vi "Process.vi"(8 "error in":errorcluster, 11 "Instrument.Framework-Template in":refnum<class "Instrument.Framework-Template.lvclass">) -> (0 "error out":errorcluster, 3 "Instrument.Framework-Template out":refnum<class "Instrument.Framework-Template.lvclass">)   [LabVIEW 2019, in "Instrument.Framework-Template.lvclass"]
doc: "---------------------------------------------------------------\nJKI State Machine Objects™\nhttp://jki.net/state-machine-objects/\nCopyright (C) 2005-2015, JKI <info@jki.net>\nALL RIGHTS RESERVED"
uses:
  Instrument.Framework-Template.lvclass
  C:/Program Files (x86)/National Instruments/LabVIEW 2019/vi.lib/JKI/JKI SMO/SMO/SMO.lvclass
  C:/Program Files (x86)/National Instruments/LabVIEW 2019/user.lib/LevyLab/Instrument Framework/Instrument/Instrument.lvclass
  Typedefs/PrivateEvents--Framework-Template.MessageToProcess.ctl
  <userlib>/LevyLab/RemoteControl/Typedefs/Message--Cluster.ctl
  Instrument.Framework-Template.lvclass/Instrument.Framework-Template.ctl
  <vilib>/JKI/JKI SMO/SMO/SMO.lvclass/SMO.ctl
  <userlib>/LevyLab/Instrument Framework/Instrument/Typedefs/Instrument.ProtectedCommands--Enum.ctl
  41410b5e-0a7b-4214-bdb2-0ee7b89dae23.vi
  <vilib>/JKI/JKI SMO/SMO/Private/ReftoDVR--SMO.vi
  <vilib>/Utility/Data Type/Get Numeric Information.vi
  <userlib>/LevyLab/Instrument Framework/Instrument/API/Instrument.sendMessageToProcess (string).vi
  <userlib>/LevyLab/Instrument Framework/Instrument Types/SCPI/Instrument.SCPI.lvclass
  <vilib>/JKI/JKI SMO/SMO/SMO.lvclass
  <userlib>/LevyLab/Instrument Framework/Instrument/Instrument.lvclass
  <userlib>/LevyLab/RemoteControl/RemoteControl.lvclass
  C:/Program Files (x86)/National Instruments/LabVIEW 2019/user.lib/LevyLab/Instrument Framework/Instrument Types/SCPI/Instrument.SCPI.lvclass
  <userlib>/LevyLab/Configuration/Debug.lvlib
panel:
  out "Status":string
  out "State History":string
  # "Instrument.Framework-Template"
  # "Framework-Template"
  # "For instructions on how to use the JKI State Machine Objects, examples and video tutorials, visit:\nhttp://jki.net/state-machine-objects/\n\nJKI State Machine Objects™\nhttp://jki.net/state-machine-objects/\nCopyright (C) 2005-2015, JKI <info@jki.net>\nALL RIGHTS RESERVED"
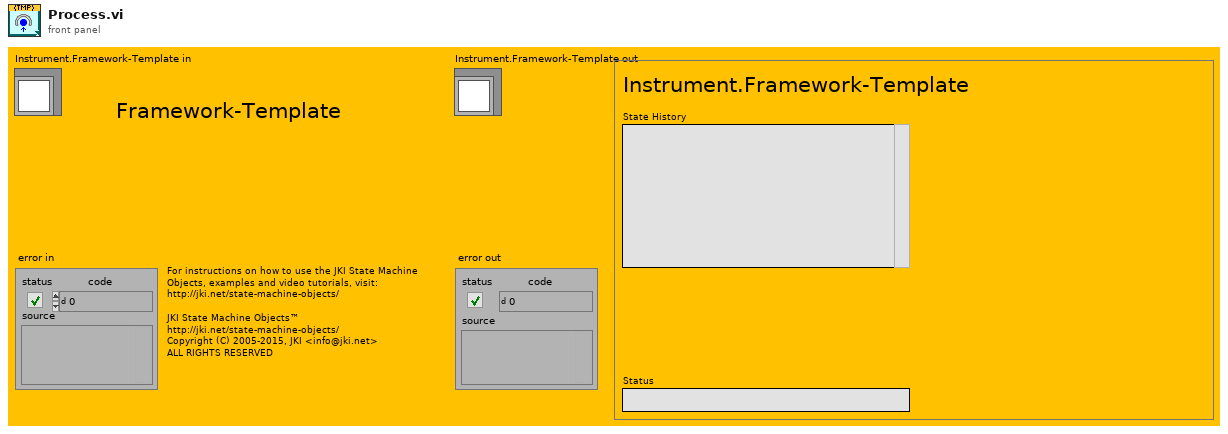
[diagram p1: front panel]
types:
  T1 = enum32{"invalid app kind", "Development System", "Run Time System", "Student Edition", "Embedded LabVIEW", "Evaluation", "Custom"}
  T2 = enum32{"Invalid", "Standard", "Closed", "Hidden", "Minimized", "Maximized"}
  T3 = typedef "Instrument.lvclass/Instrument.ProtectedCommands--Enum.ctl" = enum16{"setConfiguration", "setLogData", "setIDN", "setAll", "setAllData"}
  T4 = typedef "RemoteControl.lvclass/Message--Cluster.ctl" = cluster{"Command":string, "Data":variant, "ID":string}
  T5 = typedef "Instrument.Framework-Template.lvclass/PrivateEvents--Framework-Template.MessageToProcess.ctl" = cluster{"Message":T4}
  T6 = cluster{"Core":cluster{"Current VI Reference":refnum<vi>, "Close Panel on Exit?":bool, "Last Error":cluster{"error":errorcluster, "previous state":string, "remaining states":string}, "Shutdown?":bool}, "SelfRef":refnum<class "Instrument.Framework-Template.lvclass">, "HAL":refnum<class "HAL.lvclass">, "Running Step":i32, "sequence":string[], "MessageToProcess":T5, "UI Behavior":string, "wait":u32}
  T7 = cluster{"Current VI Reference":refnum<vi>, "Close Panel on Exit?":bool, "Last Error":cluster{"error":errorcluster, "previous state":string, "remaining states":string}, "Shutdown?":bool}
  T8 = typedef "Debug.lvlib/Attribute.Debug.lvclass/DebugBehavior.ctl" = enum16{"Normal", "Debug"}
  T9 = typedef "SMO.lvclass/Protected Events.ctl" = cluster{"StopProcesses":refnum<user-event>, "AbortProcesses":refnum<user-event>, "Config Changed":refnum<user-event>, "Dependency":refnum<user-event>}
  T10 = typedef "Instrument.Framework-Template.lvclass/Instrument.Framework-Template.getAll--Cluster.ctl" = cluster{"Levy 1":dbl, "Logger SMO":dbl, "SMO Boolean":bool, "SMO String":string}
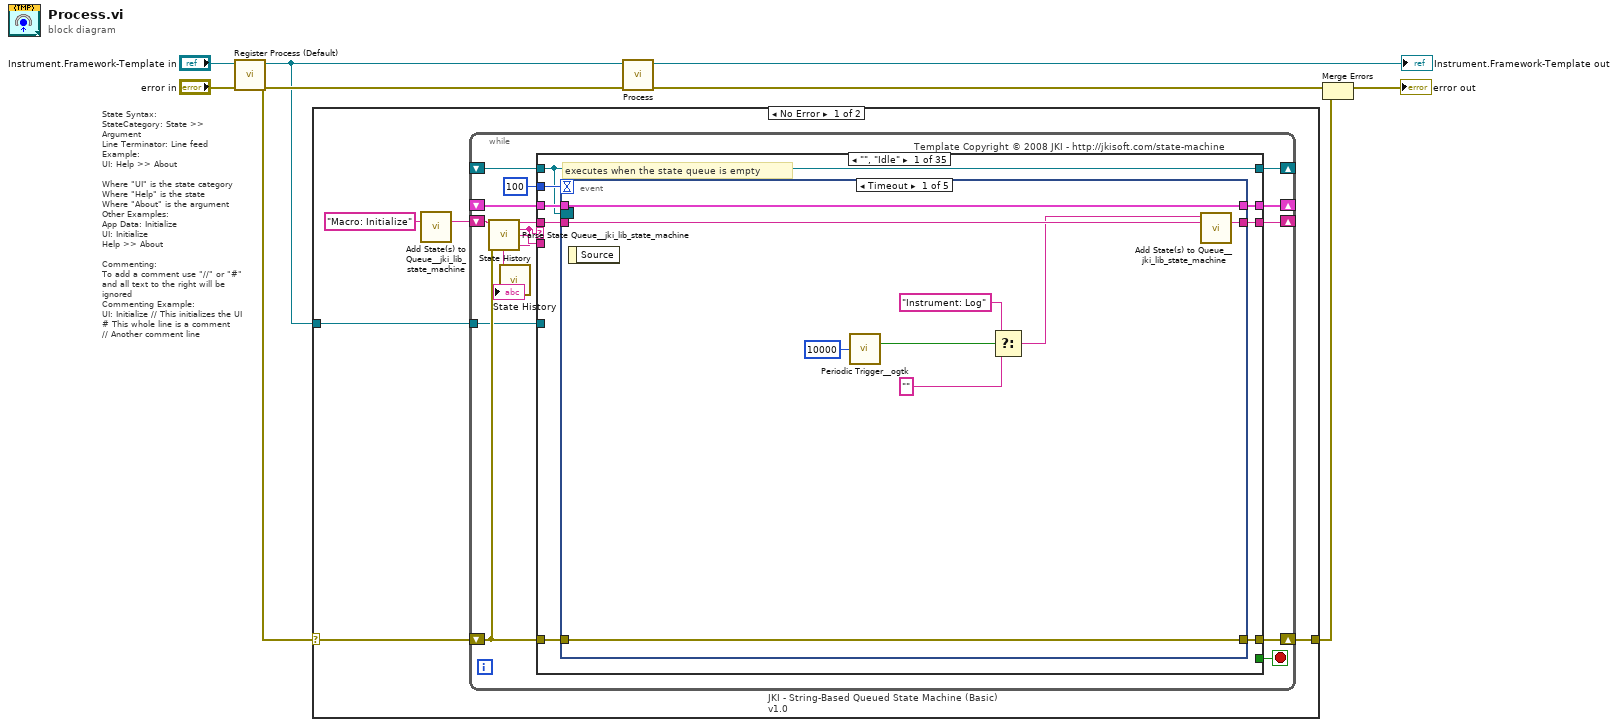
[diagram p0: block diagram]
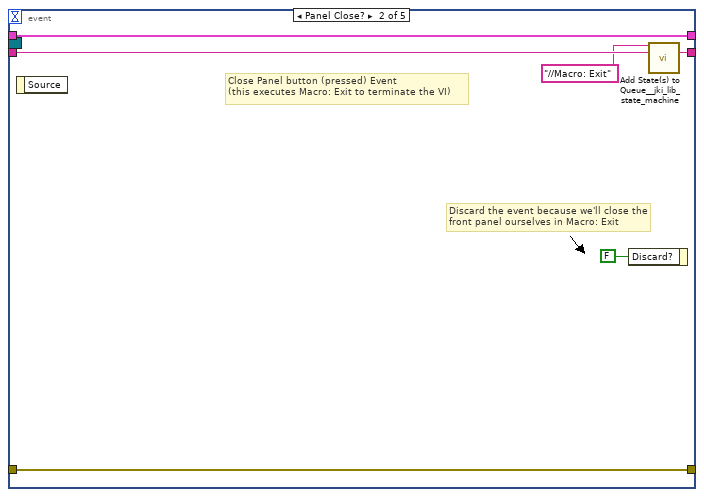
[diagram p2: hidden frame]
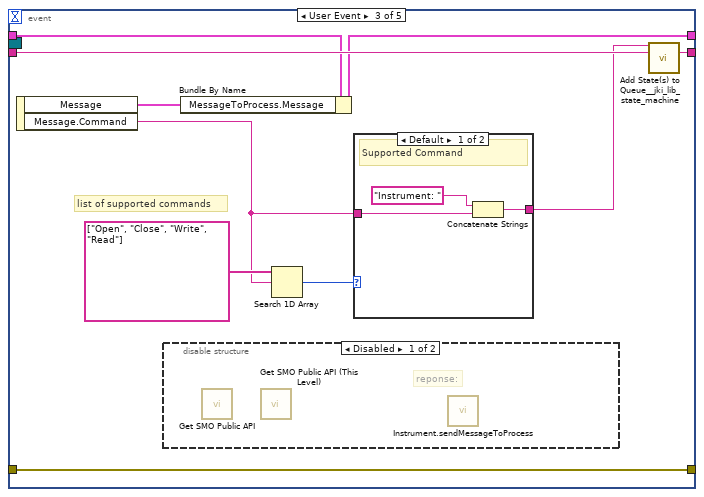
[diagram p3: hidden frame]
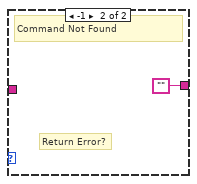
[diagram p5: hidden frame]
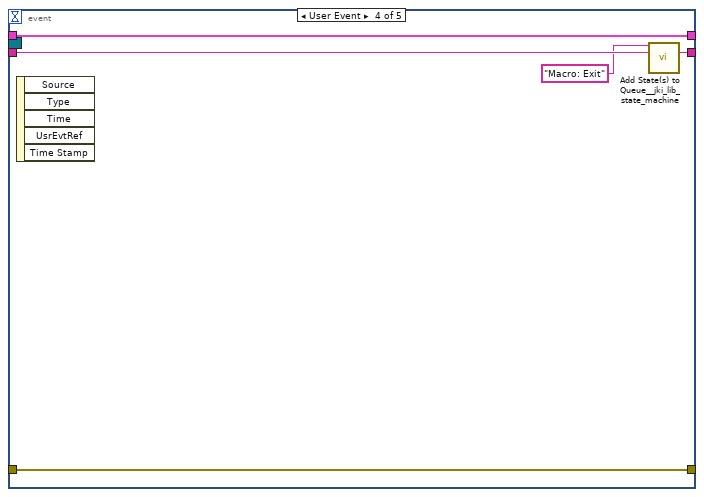
[diagram p6: hidden frame]
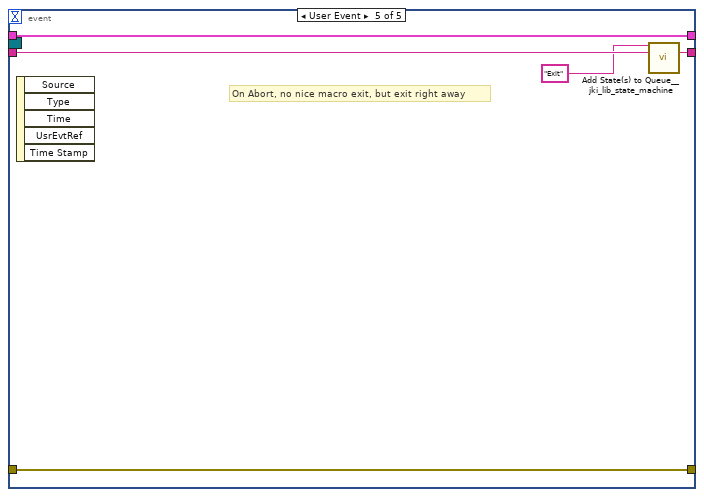
[diagram p7: hidden frame]
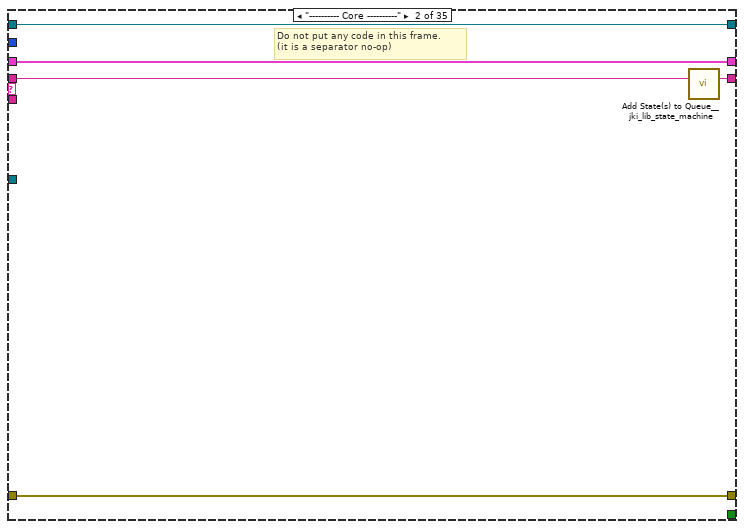
[diagram p8: hidden frame]
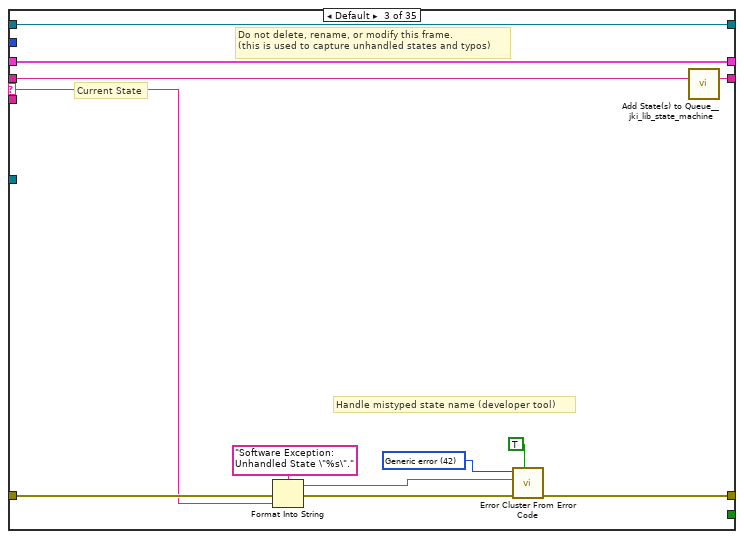
[diagram p9: hidden frame]
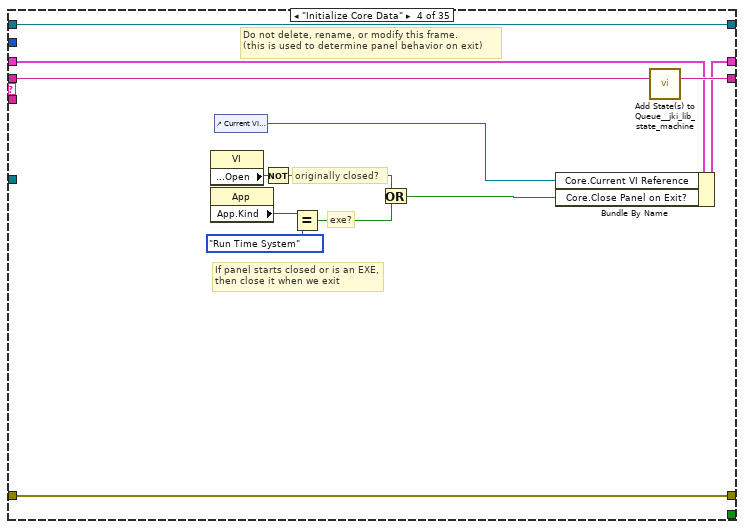
[diagram p10: hidden frame]
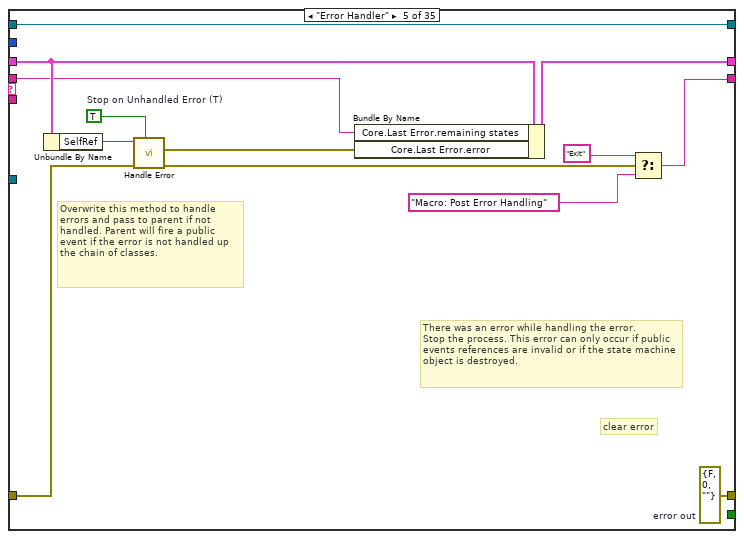
[diagram p11: hidden frame]
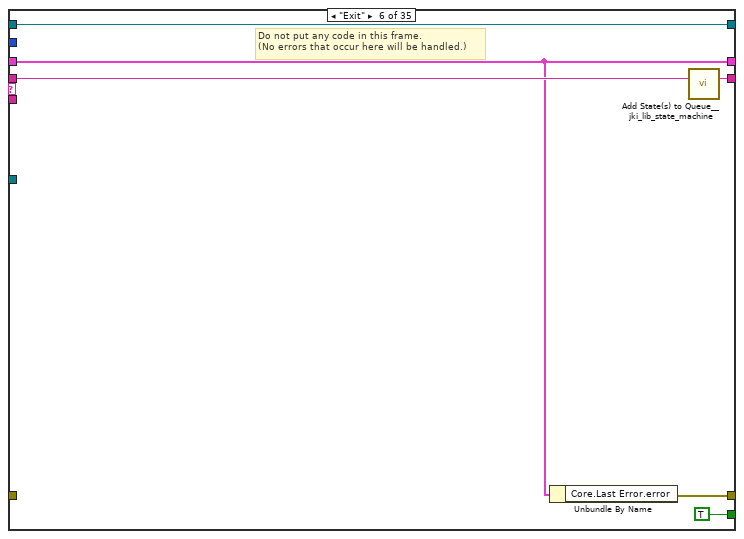
[diagram p12: hidden frame]
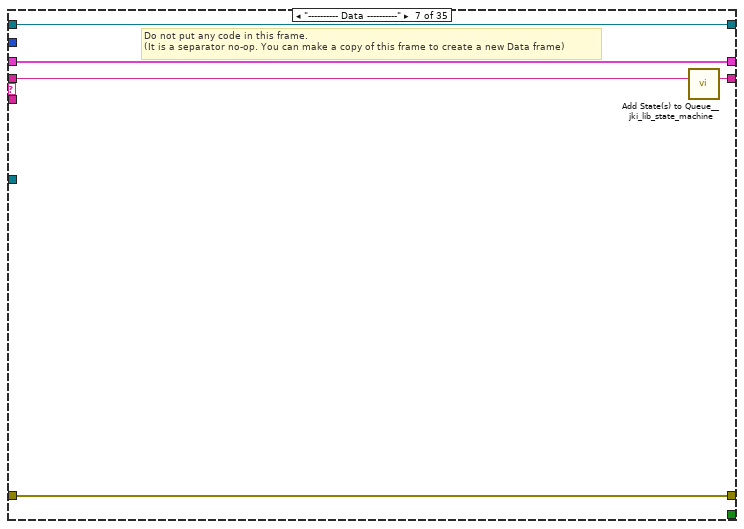
[diagram p13: hidden frame]
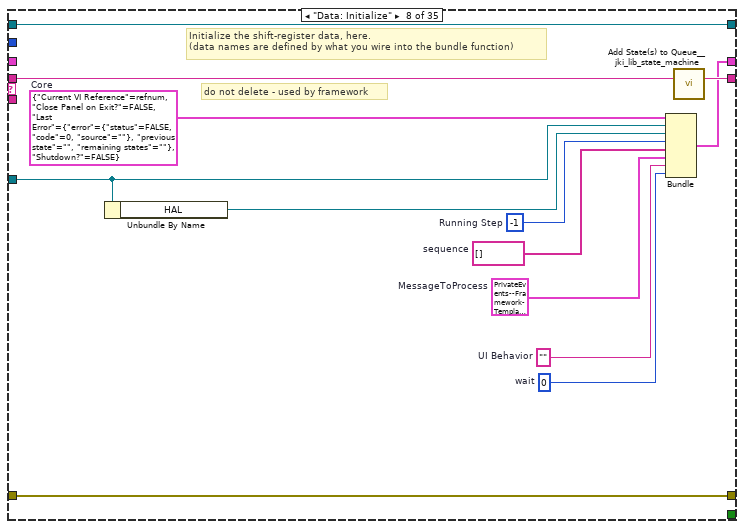
[diagram p14: hidden frame]
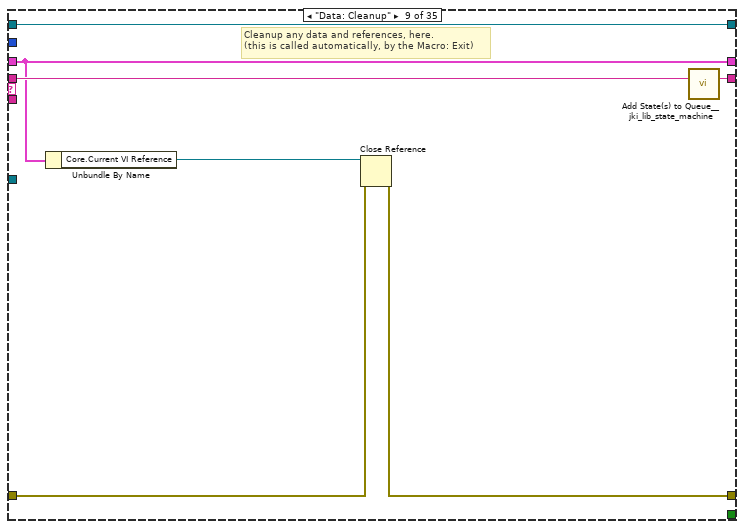
[diagram p15: hidden frame]
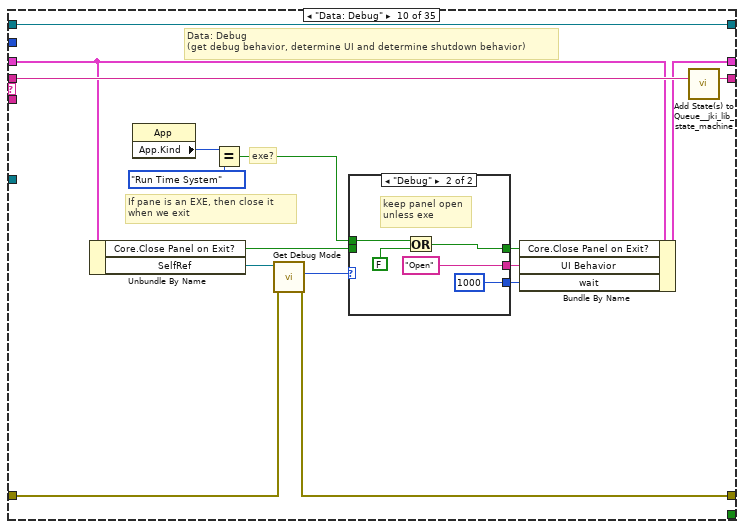
[diagram p16: hidden frame]
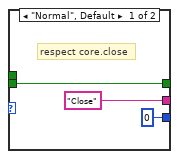
[diagram p17: hidden frame]
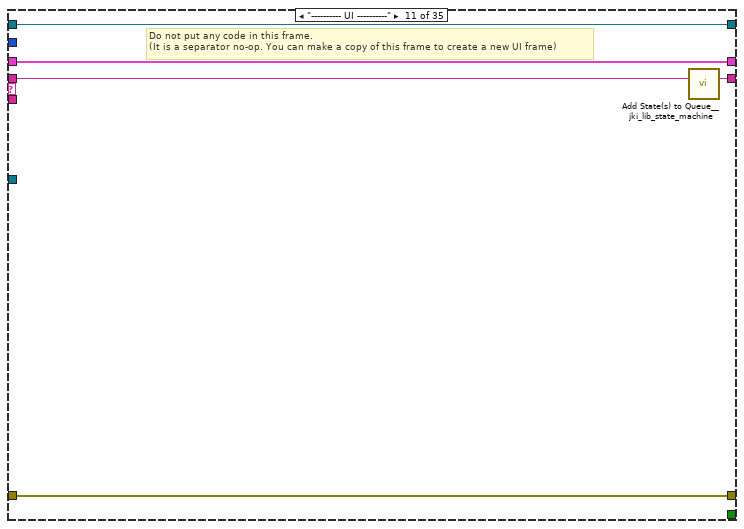
[diagram p18: hidden frame]
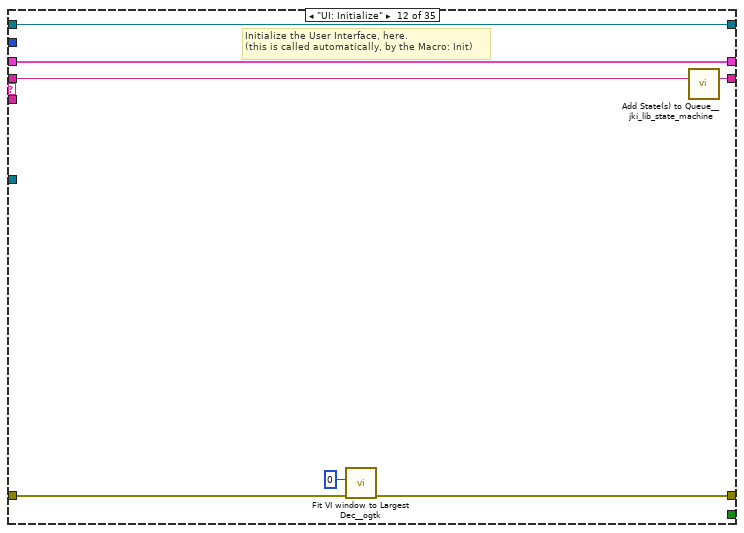
[diagram p19: hidden frame]
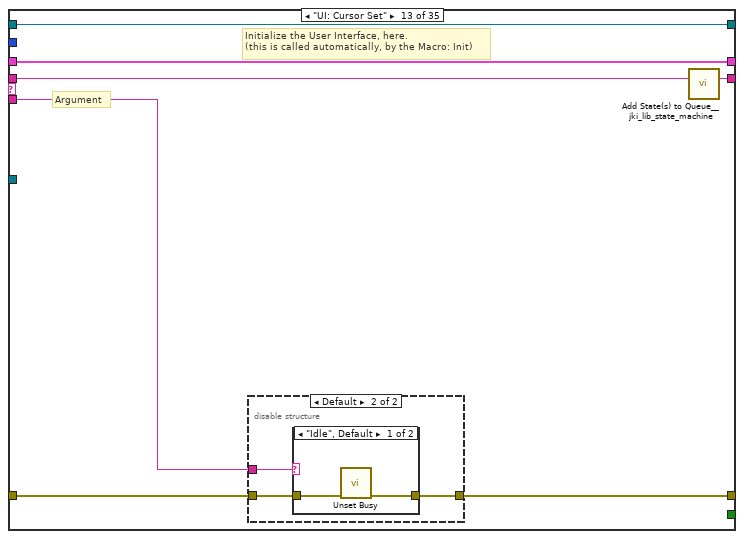
[diagram p20: hidden frame]
diagram:
  # "State Syntax:\nStateCategory: State >> Argument\nLine Terminator: Line feed\nExample:\nUI: Help >> About\n\nWhere \"UI\" is the state category\nWhere \"Help\" is the state\nWhere \"About\" is the argument\nOther Examples:\nApp Data: Initialize\nUI: Initialize\nHelp >> About\n\nCommenting:\nTo add a comment use \"//\" or \"#\" and all text to the right will be ignored\nCommenting Example:\nUI: Initialize // This initializes the UI\n# This whole line is a comment\n// Another comment line"
  n1 = call <vilib>:"Register Process (Default).vi"("error in (no error)"="error in", "SMO"="Instrument.Framework-Template in") -> ("error out"=w5:errorcluster, "SelfRef"=w4:refnum<class "Instrument.Framework-Template.lvclass">)  [unwired: 8 in]
  n2 = case shown="No Error" w5 {
    selector: w5 -> [w10 w459]
    tunnel: w4 -> [w11 _]
    tunnel: [w9 w459] -> w1
    frame No Error {
      n3 = call <vilib>:"Add State(s) to Queue__jki_lib_state_machine.vi"("State(s) in (\"\")"="Macro: Initialize") -> ("States Out"=w13:string)  [unwired: 14 in]
      n4 = while "JKI - String-Based Queued State Machine (Basic) v1.0" {
        shift-right: [w22] -> _
        shift-left: _ -> [w21]
        shift-right: [w25] -> w9
        shift-left: w10 -> [w19]
        shift-right: [w24] -> _
        shift-left: w13 -> [w26]
        tunnel: w11 -> [w18]
        shift-right: [w17] -> _
        shift-left: _ -> [w16]
        stop <- w23 stop-if-true
        # "Template Copyright © 2008 JKI - http://jkisoft.com/state-machine"
        n5 = call <vilib>:"Parse State Queue__jki_lib_state_machine.vi"("State Queue"=w26, "Error In (no error)"=w19) -> ("Remaining States"=w28:string, "Current State"=w15:string, "Arguments"=w27:string)  [unwired: 11 in]
        n6 = call <userlib>:"State History.vi"("Current State"=w15) -> ("History"=→"State History":string)  [unwired: 10 in]
        n7 = case shown="\"\", \"Idle\"" w15 {
          selector: w15 -> [_ _ w82 _ _ _ _ _ _ _ _ _ _ _ _ _ _ _ _ _ _ _ _ _ _ _ _ _ _ _ _ _ _ _ _]
          tunnel: w28 -> [w36 w80 w86 w105 w110 w124 w129 w142 w149 w165 w178 w185 w192 w208 w240 w249 w261 w282 w290 w305 w310 w321 w326 w339 w345 w353 w362 w371 w381 w390 w405 w428 w433 w439 w458]
          tunnel: w27 -> [_ _ _ _ _ _ _ _ _ _ _ _ w186 w202 _ _ _ _ _ _ _ _ _ _ _ _ _ _ _ _ _ _ _ w434 w442]
          tunnel: w21 -> [w34 w77 w84 w96 w114 w120 w126 _ w144 w152 w175 w183 w190 w204 w237 w246 w251 w272 w284 w294 w307 w318 w323 w332 w343 w348 w358 w367 w377 w386 w401 w424 w429 w435 w448]
          tunnel: [w33 w78 w88 w102 w115 w119 w127 w132 w145 w151 w176 w180 w187 w205 w238 w241 w259 w280 w288 w292 w308 w312 w324 w335 w341 w350 w354 w366 w376 w385 w395 w422 w430 w436 w450] -> w25
          tunnel: w19 -> [w32 w78 w87 w102 w116 _ w127 w132 w146 w150 w176 w179 w188 w206 w238 w241 w259 w280 w288 w292 w308 w313 w324 w329 w341 w350 w357 w365 w375 w384 w399 w417 w430 w436 w444]
          tunnel: [w35 w79 w85 w104 w106 w123 w128 w141 w148 w164 w177 w184 w191 w207 w239 w248 w260 w281 w289 w304 w309 w320 w325 w338 w344 w352 w361 w370 w380 w389 w404 w427 w432 w438 w457] -> w24
          tunnel: [_ _ _ _ _ TRUE _ _ _ _ _ _ _ _ _ _ _ _ _ _ _ _ _ _ _ _ _ _ _ _ _ _ _ _ _] -> w23
          tunnel: [w31 w77 w84 w103 w113 w120 w126 w140 w144 w153 w175 w183 w190 w204 w237 w246 w252 w273 w284 w294 w307 w318 w323 w332 w343 w349 w359 w368 w378 w387 w402 w425 w429 w435 w447] -> w22
          tunnel: 100 ("Timeout") -> [w30 _ _ _ _ _ _ _ _ _ _ _ _ _ _ _ _ _ _ _ _ _ _ _ _ _ _ _ _ _ _ _ _ _ _]
          tunnel: w18 -> [_ _ _ _ _ _ _ w133 _ _ _ _ _ _ _ _ _ _ _ _ _ _ _ _ _ _ _ _ _ _ _ _ _ _ _]
          tunnel: [w29 w76 w81 w93 w118 w121 w125 w139 w143 w163 w174 w182 w189 w201 w236 w247 w258 w279 w287 w299 w306 w319 w322 w337 w342 w351 w360 w369 w379 w388 w403 w426 w431 w437 w456] -> w17
          tunnel: w16 -> [w29 w76 w81 w93 w118 w121 w125 w139 w143 w163 w174 w182 w189 w201 w236 w247 w258 w279 w287 w299 w306 w319 w322 _ w342 w351 w360 w369 w379 w388 w403 w426 w431 w437 w456]
          frame "", "Idle" {
            # "executes when the state queue is empty"
            n8 = event shown="[0] Timeout" {
              selector: w29 -> [_ _ _ _ _]
              dyn-events: _ -> [_ _ _ _ _]
              timeout: w30 -> [_ _ _ _ _]
              tunnel: w36 -> [w45 w51 w61 w70 w75]
              tunnel: [w44 w50 w60 w69 w74] -> w35
              tunnel: w34 -> [w42 w48 w53 w67 w72]
              tunnel: [w43 w49 w59 w68 w73] -> w33
              tunnel: w32 -> [w43 w49 w59 w68 w73]
              tunnel: [w42 w48 w54 w67 w72] -> w31
              event Timeout {
                n9 = event-data() -> ()  [unwired: 1 in, 1 out]
                n10 = call <userlib>:"Periodic Trigger__ogtk.vi"("time (ms)"=u32 10000) -> ("Triggered"=w39:bool)  [unwired: 12 in, 2 out]
                n11 = Select(t="Instrument: Log", s=w39, f="") -> (s? t:f=w40:string)
                n12 = call <vilib>:"Add State(s) to Queue__jki_lib_state_machine.vi"("State(s) in Front (\"\")"=w40, "State(s) in (\"\")"=w45) -> ("States Out"=w44:string)  [unwired: 13 in]
              }
              event Panel Close? {
                # "Discard the event because we'll close the front panel ourselves in Macro: Exit"
                # "Close Panel button (pressed) Event\n(this executes Macro: Exit to terminate the VI)"
                n13 = event-data() -> ()  [unwired: 1 in, 1 out]
                n14 = event-data("Discard?"=FALSE) -> ()  [unwired: 1 in, 1 out]
                n15 = call <vilib>:"Add State(s) to Queue__jki_lib_state_machine.vi"("State(s) in Front (\"\")"="//Macro: Exit", "State(s) in (\"\")"=w51) -> ("States Out"=w50:string)  [unwired: 13 in]
              }
              event User Event {
                # "list of supported commands"
                n16 = event-data() -> ("Message"=w52:T4, "Message.Command"=w55:string)  [unwired: 1 in]
                n17 = disable-structure shown="Disabled" {
                  frame Disabled {
                    # "reponse:"
                    n18 = call-dynamic "Get SMO Public API.vi"() -> ()  [unwired: 9 in, 3 out]
                    n19 = call-dynamic "Get SMO Public API (This Level).vi"() -> ()  [unwired: 9 in, 3 out]
                    n20 = call-poly <userlib>:"Instrument.sendMessageToProcess.vi"() -> ()  [unwired: 10 in, 2 out]
                  }
                  frame Enabled {
                  }
                }
                n21 = Bundle By Name(cluster=w53, "MessageToProcess.Message"=w52) -> (w54:T6)
                n22 = Search 1D Array(1D array=string[] ["Open", "Close", "Write", "Read"], element=w55) -> (index of element=w58:i32)  [unwired: 1 in]
                n23 = case shown="Default" w58 {
                  tunnel: [w64 ""] -> w56
                  tunnel: w55 -> [w63 _]
                  frame Default {
                    # "Supported Command"
                    n24 = Concatenate Strings("Instrument: ", w63) -> (w64:string)
                  }
                  frame -1 {
                    # "Return Error?"
                    # "Command Not Found"
                  }
                }
                n25 = call <vilib>:"Add State(s) to Queue__jki_lib_state_machine.vi"("State(s) in Front (\"\")"=w56, "State(s) in (\"\")"=w61) -> ("States Out"=w60:string)  [unwired: 13 in]
              }
              event User Event {
                n26 = event-data() -> ()  [unwired: 1 in, 5 out]
                n27 = call <vilib>:"Add State(s) to Queue__jki_lib_state_machine.vi"("State(s) in Front (\"\")"="Macro: Exit", "State(s) in (\"\")"=w70) -> ("States Out"=w69:string)  [unwired: 13 in]
              }
              event User Event {
                # "On Abort, no nice macro exit, but exit right away"
                n28 = event-data() -> ()  [unwired: 1 in, 5 out]
                n29 = call <vilib>:"Add State(s) to Queue__jki_lib_state_machine.vi"("State(s) in Front (\"\")"="Exit", "State(s) in (\"\")"=w75) -> ("States Out"=w74:string)  [unwired: 13 in]
              }
            }
          }
          frame "---------- Core ----------" {
            # "Do not put any code in this frame.\n(it is a separator no-op)"
            n30 = call <vilib>:"Add State(s) to Queue__jki_lib_state_machine.vi"("State(s) in (\"\")"=w80) -> ("States Out"=w79:string)  [unwired: 14 in]
          }
          frame Default {
            w91 = 42 items=["No error", "Argument error", "Memory is full", "Out of zone", "End of file", "File already open", "Generic file I/O error", "File not found", "File permission error", "Disk is full", "Duplicate path", "Too many files open", "System feature not enabled", "Resource file not found", "Cannot add resource", "Resource not found", "Image not found", "Image memory error", "Pen does not exist", "Config type invalid", "Config token not found", "Config parse error", "Config memory error", "Bad external code format", "Bad external code offset", "External code not present", "Null window", "Destroy window error", "Null menu", "Print aborted", "Bad print record", "Print driver error", "Windows error during printing", "Memory error during printing", "Print dialog error", "Generic print error", "Invalid device refnum", "Device not found", "Device parameter error", "Device unit error", "Cannot open device", "Device call aborted", "Generic error", "Cancelled by user", "Object ID too low", "Object ID too high", "Object not in heap", "Unknown heap", "Unknown object (invalid DefProc)", "Unknown object (DefProc not in table)", "Message out of range", "Invalid (null) method", "Unknown message", "Manager call not supported", "Bad address", "Network operation in progress", "Network operation timed out", "Connection is busy", "Network attribute not supported", "Network error", "Address in use", "System out of memory", "Connection aborted", "Connection refused", "Not connected", "Already connected", "Connection closed", "Initialization error (interapplication manager)", "Bad occurrence", "Wait on unbound occurrence handler", "Occurrence queue overflow", "Datalog type conflict", "Unused", "Unrecognized type (interapplication manager)", "Memory corrupt", "Failed to make temporary DLL", "Old CIN version", "Drag socket not found", "Failed to load drop-object", "Failed to register OLE object", "Failed to release OLE object", "Format specifier type mismatch", "Unknown format specifier", "Too few format specifiers", "Too many format specifiers", "Scan failed", "Newer CIN version", "Error converting to variant", "Runtime menu error", "Password tampered", "Variant attribute not found", "Incompatible variant data type", "Event data is not available", "Event Store is not present", "Occurrence is not found", "Event Queue is not created", "Event info is not available", "Refnum passed is NULL", "Error retrieving Class GUID", "Error retrieving CoClass GUID", "Error retrieving TypeLib GUID.", "Bad built application magic bytes.", "Specific driver is different from the specific driver associated with the Logical Name.", "There is no session opened to the class driver.", "Max Error", "MAX - Error with config objects", "MAX - Error loading configuration", "MAX - Group not supported"]
            # "Current State"
            # "Do not delete, rename, or modify this frame.\n(this is used to capture unhandled states and typos)"
            # "Handle mistyped state name (developer tool)"
            n31 = Format Into String(format string="Software Exception: Unhandled State \"%s\"." ("message"), error in=w87, w82) -> (resulting string=w90:string, error out=w89:errorcluster)  [unwired: 1 in]
            n32 = call <vilib>:"Error Cluster From Error Code.vi"("show call chain? (False)"=TRUE, "error in (no error)"=w89, "error message (\"\")"=w90, "error code (0)"=w91) -> ("error out"=w88:errorcluster)  [unwired: 5 in]
            n33 = call <vilib>:"Add State(s) to Queue__jki_lib_state_machine.vi"("State(s) in (\"\")"=w86) -> ("States Out"=w85:string)  [unwired: 14 in]
          }
          frame "Initialize Core Data" {
            # "Do not delete, rename, or modify this frame.\n(this is used to determine panel behavior on exit)"
            # "originally closed?"
            # "exe?"
            # "If panel starts closed or is an EXE, then close it when we exit"
            n34 = property class="VI"() -> ("Front Panel.Open"=w101:bool)  [unwired: 2 in, 2 out]
            n35 = property class="App"() -> ("App.Kind"=w100:T1)  [unwired: 2 in, 2 out]
            n36 = control-ref of="Current VI Reference"() -> (w94:refnum<vi>)
            n37 = Not(x=w101) -> (.not. x?=w98:bool)
            n38 = Equal?(x=w100, y=T1."Run Time System" ("Application:Kind")) -> (x = y?=w97:bool)
            n39 = Or(x=w98, y=w97) -> (x .or. y?=w95:bool)
            n40 = Bundle By Name(cluster=w96, "Core.Current VI Reference"=w94, "Core.Close Panel on Exit?"=w95) -> (w103:T6)
            n41 = call <vilib>:"Add State(s) to Queue__jki_lib_state_machine.vi"("State(s) in (\"\")"=w105) -> ("States Out"=w104:string)  [unwired: 14 in]
          }
          frame "Error Handler" {
            w111 = TRUE  # Stop on Unhandled Error (T)
            w115 = errorcluster {"status"=FALSE, "code"=0, "source"=""}  # error out
            # "clear error"
            # "There was an error while handling the error.\nStop the process. This error can only occur if public events references are invalid or if the state machine object is destroyed."
            # "Overwrite this method to handle errors and pass to parent if not handled. Parent will fire a public event if the error is not handled up the chain of classes."
            n42 = Unbundle By Name(w114) -> ("SelfRef"=w117:refnum<class "Instrument.Framework-Template.lvclass">)
            n43 = call-dynamic "Handle Error.vi"("Stop on Unhandled Error (T)"=w111, "error in"=w116, "SMO"=w117) -> ("handling error"=w107:errorcluster, "Unhandled error"=w112:errorcluster)  [unwired: 6 in, 1 out]
            n44 = Bundle By Name(cluster=w114, "Core.Last Error.remaining states"=w110, "Core.Last Error.error"=w112) -> (w113:T6)
            n45 = Select(t="Exit", s=w107, f="Macro: Post Error Handling") -> (s? t:f=w106:string)
          }
          frame "Exit" {
            # "Do not put any code in this frame.\n(No errors that occur here will be handled.)"
            n46 = Unbundle By Name(w120) -> ("Core.Last Error.error"=w119:errorcluster)
            n47 = call <vilib>:"Add State(s) to Queue__jki_lib_state_machine.vi"("State(s) in (\"\")"=w124) -> ("States Out"=w123:string)  [unwired: 14 in]
          }
          frame "---------- Data ----------" {
            # "Do not put any code in this frame.\n(It is a separator no-op. You can make a copy of this frame to create a new Data frame)"
            n48 = call <vilib>:"Add State(s) to Queue__jki_lib_state_machine.vi"("State(s) in (\"\")"=w129) -> ("States Out"=w128:string)  [unwired: 14 in]
          }
          frame "Data: Initialize" {
            w130 = u32 0  # wait
            w131 = ""  # UI Behavior
            w135 = T5 {"Message"={"Command"="", "Data"=variant(string ""), "ID"=""}}  # MessageToProcess
            w136 = string[] []  # sequence
            w137 = -1  # Running Step
            w138 = T7 {"Current VI Reference"=refnum, "Close Panel on Exit?"=FALSE, "Last Error"={"error"={"status"=FALSE, "code"=0, "source"=""}, "previous state"="", "remaining states"=""}, "Shutdown?"=FALSE}  # Core
            # "do not delete - used by framework"
            # "Initialize the shift-register data, here.\n(data names are defined by what you wire into the bundle function)"
            n49 = Unbundle By Name(w133) -> ("HAL"=w134:refnum<class "HAL.lvclass">)
            n50 = Bundle("Core"=w138, "SelfRef"=w133, "HAL"=w134, "Running Step"=w137, "sequence"=w136, "MessageToProcess"=w135, "UI Behavior"=w131, "wait"=w130) -> (w140:T6)  [unwired: 1 in]
            n51 = call <vilib>:"Add State(s) to Queue__jki_lib_state_machine.vi"("State(s) in (\"\")"=w142) -> ("States Out"=w141:string)  [unwired: 14 in]
          }
          frame "Data: Cleanup" {
            # "Cleanup any data and references, here.\n(this is called automatically, by the Macro: Exit)"
            n52 = Unbundle By Name(w144) -> ("Core.Current VI Reference"=w147:refnum<vi>)
            n53 = Close Reference(reference=w147, error in (no error)=w146) -> (error out=w145:errorcluster)
            n54 = call <vilib>:"Add State(s) to Queue__jki_lib_state_machine.vi"("State(s) in (\"\")"=w149) -> ("States Out"=w148:string)  [unwired: 14 in]
          }
          frame "Data: Debug" {
            # "exe?"
            # "If pane is an EXE, then close it when we exit"
            # "Data: Debug\n(get debug behavior, determine UI and determine shutdown behavior)"
            n55 = Unbundle By Name(w152) -> ("Core.Close Panel on Exit?"=w155:bool, "SelfRef"=w162:refnum<class "Instrument.Framework-Template.lvclass">)
            n56 = property class="App"() -> ("App.Kind"=w158:T1)  [unwired: 2 in, 2 out]
            n57 = Equal?(x=w158, y=T1."Run Time System" ("Application:Kind")) -> (x = y?=w154:bool)
            n58 = call <userlib>:"Get Debug Mode.vi"("error in (no error)"=w150, "SMO"=w162) -> ("error out"=w151:errorcluster, "Behavior"=w161:T8)  [unwired: 7 in, 1 out]
            n59 = case shown="\"Debug\"" w161 {
              tunnel: ["Close" "Open"] -> w160
              tunnel: [u32 0 ("wait") u32 1000 ("wait")] -> w159
              tunnel: [w166 w169] -> w156
              tunnel: w155 -> [w166 _]
              tunnel: w154 -> [_ w171]
              frame "Normal", Default {
                # "respect core.close"
              }
              frame "Debug" {
                # "keep panel open\nunless exe"
                n60 = Or(x=w171, y=FALSE) -> (x .or. y?=w169:bool)
              }
            }
            n61 = Bundle By Name(cluster=w152, "Core.Close Panel on Exit?"=w156, "UI Behavior"=w160, "wait"=w159) -> (w153:T6)
            n62 = call <vilib>:"Add State(s) to Queue__jki_lib_state_machine.vi"("State(s) in (\"\")"=w165) -> ("States Out"=w164:string)  [unwired: 14 in]
          }
          frame "---------- UI ----------" {
            # "Do not put any code in this frame.\n(It is a separator no-op. You can make a copy of this frame to create a new UI frame)"
            n63 = call <vilib>:"Add State(s) to Queue__jki_lib_state_machine.vi"("State(s) in (\"\")"=w178) -> ("States Out"=w177:string)  [unwired: 14 in]
          }
          frame "UI: Initialize" {
            # "Initialize the User Interface, here.\n(this is called automatically, by the Macro: Init)"
            n64 = call <userlib>:"Fit VI window to Largest Dec__ogtk.vi"("error in (no error)"=w179, "border spacing (2 px)"=0) -> ("error out"=w180:errorcluster)  [unwired: 4 in, 1 out]
            n65 = call <vilib>:"Add State(s) to Queue__jki_lib_state_machine.vi"("State(s) in (\"\")"=w185) -> ("States Out"=w184:string)  [unwired: 14 in]
          }
          frame "UI: Cursor Set" {
            # "Argument"
            # "Initialize the User Interface, here.\n(this is called automatically, by the Macro: Init)"
            n66 = disable-structure shown="Default" {
              disable-tunnel: w188 -> [w193 w196]
              disable-tunnel: [w193 w195] -> w187
              disable-tunnel: w186 -> [_ w194]
              frame condition #0 {
              }
              frame condition #1 (active) {
                n67 = case shown="\"Idle\", Default" w194 {
                  tunnel: w196 -> [w198 w200]
                  tunnel: [w197 w199] -> w195
                  frame "Idle", Default {
                    n68 = call <vilib>:"Unset Busy.vi"("error in (no error)"=w198) -> ("error out"=w197:errorcluster)  [unwired: 10 in]
                  }
                  frame "Busy" {
                    n69 = call <vilib>:"Set Busy.vi"("error in (no error)"=w200) -> ("error out"=w199:errorcluster)  [unwired: 9 in, 1 out]
                  }
                }
              }
            }
            n70 = call <vilib>:"Add State(s) to Queue__jki_lib_state_machine.vi"("State(s) in (\"\")"=w192) -> ("States Out"=w191:string)  [unwired: 14 in]
          }
          frame "UI: Front Panel State" {
            # "Argument"
            # "Set Front Panel Open or Closed\n(Usage: \"UI: Front Panel State >> Open|Close\")"
            n71 = Unbundle By Name(w204) -> ("Core.Current VI Reference"=w203:refnum<vi>)
            n72 = disable-structure shown="TARGET_TYPE==RT" {
              disable-tunnel: w206 -> [w212 w235]
              disable-tunnel: [w211 w235] -> w205
              disable-tunnel: w203 -> [w210 _]
              disable-tunnel: w202 -> [w209 _]
              frame condition #0 (active) {
                n73 = case shown="\"Close\"" w209 {
                  tunnel: w212 -> [w216 w229]
                  tunnel: [w218 w230] -> w211
                  tunnel: w210 -> [w217 w227]
                  frame "Open", Default {
                    n74 = property class="VI"(reference=w217, error in=w216) -> (reference out=w214:refnum<vi>, error out=w215:errorcluster, "FP.State"=w213:T2)
                    n75 = case shown="\"Closed\"" w213 {
                      tunnel: [w221 w224] -> w218
                      tunnel: w215 -> [w220 w224]
                      tunnel: w214 -> [w219 _]
                      frame "Closed" {
                        n76 = invoke class="VI" method="FP.Open"(reference=w219, error in=w220, "Activate"=TRUE, "State"=T2."Standard") -> (error out=w221:errorcluster)  [unwired: 1 in, 4 out]
                      }
                      frame Default {
                      }
                    }
                  }
                  frame "Close" {
                    n77 = property class="VI"(reference=w227, error in=w229) -> (reference out=w226:refnum<vi>, error out=w228:errorcluster, "FP.State"=w225:T2)
                    n78 = case shown="Default" w225 {
                      tunnel: [w231 w234] -> w230
                      tunnel: w228 -> [w231 w233]
                      tunnel: w226 -> [_ w232]
                      frame "Invalid", "Closed" {
                      }
                      frame Default {
                        n79 = invoke class="VI" method="FP.Close"(reference=w232, error in=w233) -> (error out=w234:errorcluster)  [unwired: 1 in, 2 out]
                      }
                    }
                  }
                }
              }
              frame condition #1 {
              }
            }
            n80 = call <vilib>:"Add State(s) to Queue__jki_lib_state_machine.vi"("State(s) in (\"\")"=w208) -> ("States Out"=w207:string)  [unwired: 14 in]
          }
          frame "---------- Macro ----------" {
            # "Do not put any code in this frame.\n(It is a separator no-op. You can make a copy of this frame to create a new Macro frame)"
            n81 = call <vilib>:"Add State(s) to Queue__jki_lib_state_machine.vi"("State(s) in (\"\")"=w240) -> ("States Out"=w239:string)  [unwired: 14 in]
          }
          frame "Macro: Initialize" {
            # "Initialization Macro\n(This is called once, when the VI starts)"
            n82 = call <vilib>:"Add State(s) to Queue__jki_lib_state_machine.vi"("State(s) in Front (\"\")"="Data: Initialize\nInitialize Core Data\nEvents: Register", "State(s) in (\"\")"="Process: Sync", "State(s) at Back (\"\")"="UI: Initialize\nUI: Front Panel State >> Close\nInstrument: Open\nMacro: Debug") -> ("States Out"=w244:string)  [unwired: 12 in]
            n83 = call <vilib>:"Add State(s) to Queue__jki_lib_state_machine.vi"("State(s) in Front (\"\")"=w244, "State(s) in (\"\")"=w249) -> ("States Out"=w248:string)  [unwired: 13 in]
          }
          frame "Macro: Post Error Handling" {
            # "Clear Last Error?"
            n84 = Unbundle By Name(w251) -> ("Core.Last Error.remaining states"=w253:string, "Core.Shutdown?"=w254:bool)
            n85 = Unbundle By Name(w251) -> ("Core.Last Error.error"=w257:errorcluster)
            n86 = case shown="False" FALSE {
              tunnel: w257 -> [w265 _]
              tunnel: [w265 _] -> w256
              frame False {
              }
              frame True {
              }
            }
            n87 = case shown="False" w254 {
              tunnel: w253 -> [w262 w264]
              tunnel: [w262 w263] -> w250
              frame False {
                # "These are the remaining states (at the moment the error occured). States can be altered according to business logic."
                # "NOT SHUTTING DOWN"
              }
              frame True {
                # "Developer can decide to alter the states but should be aware that during the shutdown process, there are certain states that must be run for the SMO to properly shut itself (and this process) down. As such, one can add states to perform additional clean-ups, but should append the remaining state to be executed."
                # "SHUTTING DOWN"
                n88 = call <vilib>:"Add State(s) to Queue__jki_lib_state_machine.vi"("State(s) in (\"\")"=w264) -> ("States Out"=w263:string)  [unwired: 14 in]
              }
            }
            n89 = Bundle By Name(cluster=w251, "Core.Last Error.error"=w256) -> (w252:T6)
            n90 = call <vilib>:"Add State(s) to Queue__jki_lib_state_machine.vi"("State(s) in Front (\"\")"=w250, "State(s) in (\"\")"=w261) -> ("States Out"=w260:string)  [unwired: 13 in]
          }
          frame "Macro: Run Sequence" {
            # "0,1,2,3,4,"
            # "5"
            # "Do not put any code in this frame.\n(It is a separator no-op. You can make a copy of this frame to create a new Macro frame)"
            n91 = Unbundle By Name(w272) -> ("sequence"=w268:string[], "Running Step"=w266:i32)
            n92 = Array Size(array=w268) -> (size(s)=w278:i32)
            n93 = Index Array(array=w268, index=w266) -> (element=w267:string)
            n94 = Greater Or Equal?(x=w278, y=w266) -> (x >= y?=w270:bool)
            n95 = Select(t=-1 ("Running Step"), s=w270, f=w266) -> (s? t:f=w277:i32)
            n96 = Bundle By Name(cluster=w272, "Running Step"=w277) -> (w273:T6)
            n97 = Select(t="Sequence: Status >> ...", s=w270, f="Idle //Check Event Structure\nMacro: Run Sequence" ("State(s) at Back (\"\")")) -> (s? t:f=w269:string)
            n98 = call <vilib>:"Add State(s) to Queue__jki_lib_state_machine.vi"("State(s) in Front (\"\")"=w267, "State(s) at Back (\"\")"=w269) -> ("States Out"=w271:string)  [unwired: 13 in]
            n99 = call <vilib>:"Add State(s) to Queue__jki_lib_state_machine.vi"("State(s) in Front (\"\")"=w271, "State(s) in (\"\")"=w282) -> ("States Out"=w281:string)  [unwired: 13 in]
          }
          frame "Macro: Debug" {
            n100 = Unbundle By Name(w284) -> ("UI Behavior"=w286:string)
            n101 = Format Into String(format string="Data: Debug\nUI: Front Panel State >> %s\n//UI: Wait" ("State(s) in Front (\"\")"), w286) -> (resulting string=w283:string)  [unwired: 2 in, 1 out]
            n102 = call <vilib>:"Add State(s) to Queue__jki_lib_state_machine.vi"("State(s) in Front (\"\")"=w283, "State(s) in (\"\")"=w290) -> ("States Out"=w289:string)  [unwired: 13 in]
          }
          frame "Macro: Exit" {
            # "Exit Macro\n(This is called once, when the VI exits)"
            n103 = Unbundle By Name(w294) -> ("Core.Close Panel on Exit?"=w303:bool)
            n104 = Select(t="UI: Front Panel State >> Close", s=w303, f="") -> (s? t:f=w301:string)
            n105 = call <vilib>:"Add State(s) to Queue__jki_lib_state_machine.vi"("State(s) in Front (\"\")"="Data: Cleanup\nEvents: Unregister", "State(s) in (\"\")"="Process: Sync", "State(s) at Back (\"\")"="Exit") -> ("States Out"=w296:string)  [unwired: 12 in]
            n106 = call <vilib>:"Add State(s) to Queue__jki_lib_state_machine.vi"("State(s) in Front (\"\")"="Instrument: Close", "State(s) in (\"\")"=w301, "State(s) at Back (\"\")"=w296) -> ("States Out"=w300:string)  [unwired: 12 in]
            n107 = call <vilib>:"Add State(s) to Queue__jki_lib_state_machine.vi"("State(s) in Front (\"\")"=w300, "State(s) in (\"\")"=w305) -> ("States Out"=w304:string)  [unwired: 13 in]
          }
          frame "---------- Process ----------" {
            # "Template Separator\n(You can make a copy of, or modify, this frame)"
            n108 = call <vilib>:"Add State(s) to Queue__jki_lib_state_machine.vi"("State(s) in (\"\")"=w310) -> ("States Out"=w309:string)  [unwired: 14 in]
          }
          frame "Process: Sync" {
            n109 = Unbundle By Name(w318) -> ("SelfRef"=w314:refnum<class "Instrument.Framework-Template.lvclass">)
            n110 = call <vilib>:"WaitOnProcessSync.vi"("error in (no error)"=w313, "SMO"=w314) -> ("error out"=w312:errorcluster, "Don't run?"=w317:bool)  [unwired: 7 in, 1 out]
            n111 = Select(t="Data: Cleanup\nEvents: Unregister\nExit", s=w317, f="") -> (s? t:f=w311:string)
            n112 = call <vilib>:"Add State(s) to Queue__jki_lib_state_machine.vi"("State(s) in Front (\"\")"=w311, "State(s) in (\"\")"=w321) -> ("States Out"=w320:string)  [unwired: 13 in]
          }
          frame "---------- Events ----------" {
            # "Template Separator\n(You can make a copy of, or modify, this frame)"
            n113 = call <vilib>:"Add State(s) to Queue__jki_lib_state_machine.vi"("State(s) in (\"\")"=w326) -> ("States Out"=w325:string)  [unwired: 14 in]
          }
          frame "Events: Register" {
            n114 = Unbundle By Name(w332) -> ("SelfRef"=w333:refnum<class "Instrument.Framework-Template.lvclass">)
            n115 = call <vilib>:"GetProtectedEvents.vi"("SMO"=w333) -> ("error out"=w331:errorcluster, "SMO Protected Events"=w336:T9, "SMO out"=w330:refnum<class "Instrument.Framework-Template.lvclass">)  [unwired: 8 in]
            n116 = call "Instrument-Template.GetPrivateEvents.vi"("Instrument.Framework-Template in"=w330) -> ("error out"=w327:errorcluster, "Framework-Template Private Events"=w328:cluster{"MessageToProcess":refnum<user-event>})  [unwired: 8 in, 1 out]
            n117 = register-events(w336, w328) -> (reference out=w337:refnum<event-registration>, error out=w334:errorcluster)  [unwired: 2 in]
            n118 = Merge Errors(w334, w327, w331, w329) -> (w335:errorcluster)
            n119 = call <vilib>:"Add State(s) to Queue__jki_lib_state_machine.vi"("State(s) in (\"\")"=w339) -> ("States Out"=w338:string)  [unwired: 14 in]
          }
          frame "Events: Unregister" {
            n120 = Unregister For Events(event registration refnum=w342, error in=w341) -> (error out=w340:errorcluster)
            n121 = call <vilib>:"Clear Errors.vi"("error in (no error)"=w340) -> ()  [unwired: 5 in, 2 out]
            n122 = call <vilib>:"Add State(s) to Queue__jki_lib_state_machine.vi"("State(s) in (\"\")"=w345) -> ("States Out"=w344:string)  [unwired: 14 in]
          }
          frame "---------- Instrument ----------" {
            n123 = Unbundle By Name(w348) -> ("SelfRef"=w346:refnum<class "Instrument.Framework-Template.lvclass">, "HAL"=w347:refnum<class "HAL.lvclass">)
            n124 = Bundle By Name(cluster=w348, "SelfRef"=w346, "HAL"=w347) -> (w349:T6)
            n125 = call <vilib>:"Add State(s) to Queue__jki_lib_state_machine.vi"("State(s) in (\"\")"=w353) -> ("States Out"=w352:string)  [unwired: 14 in]
          }
          frame "Instrument: Open" {
            n126 = Unbundle By Name(w358) -> ("SelfRef"=w356:refnum<class "Instrument.Framework-Template.lvclass">)
            n127 = call-dynamic "Open Hardware.vi"("error in (no error)"=w357, "Instrument in"=w356) -> ("error out"=w354:errorcluster, "Instrument out"=w355:refnum<class "Instrument.Framework-Template.lvclass">)  [unwired: 8 in]
            n128 = Bundle By Name(cluster=w358, "SelfRef"=w355) -> (w359:T6)
            n129 = call <vilib>:"Add State(s) to Queue__jki_lib_state_machine.vi"("State(s) in (\"\")"=w362) -> ("States Out"=w361:string)  [unwired: 14 in]
          }
          frame "Instrument: Write" {
            n130 = Unbundle By Name(w367) -> ("SelfRef"=w364:refnum<class "Instrument.Framework-Template.lvclass">)
            n131 = call-dynamic "Write Hardware.vi"("error in (no error)"=w365, "Instrument in"=w364) -> ("error out"=w366:errorcluster, "Instrument out"=w363:refnum<class "Instrument.Framework-Template.lvclass">)  [unwired: 8 in]
            n132 = Bundle By Name(cluster=w367, "SelfRef"=w363) -> (w368:T6)
            n133 = call <vilib>:"Add State(s) to Queue__jki_lib_state_machine.vi"("State(s) in (\"\")"=w371) -> ("States Out"=w370:string)  [unwired: 14 in]
          }
          frame "Instrument: Read" {
            n134 = Unbundle By Name(w377) -> ("SelfRef"=w373:refnum<class "Instrument.Framework-Template.lvclass">)
            n135 = call-dynamic "Read Hardware.vi"("error in (no error)"=w375, "Instrument in"=w373) -> ("error out"=w376:errorcluster, "response"=w374:string, "Instrument out"=w372:refnum<class "Instrument.Framework-Template.lvclass">)  [unwired: 7 in]
            n136 = Bundle By Name(cluster=w377, "SelfRef"=w372, "MessageToProcess.Message.Data"=w374) -> (w378:T6)
            n137 = call <vilib>:"Add State(s) to Queue__jki_lib_state_machine.vi"("State(s) in (\"\")"=w381) -> ("States Out"=w380:string)  [unwired: 14 in]
          }
          frame "Instrument: Close" {
            n138 = Unbundle By Name(w386) -> ("SelfRef"=w383:refnum<class "Instrument.Framework-Template.lvclass">)
            n139 = call-dynamic "Close Hardware.vi"("error in (no error)"=w384, "Instrument in"=w383) -> ("error out"=w385:errorcluster, "Instrument out"=w382:refnum<class "Instrument.Framework-Template.lvclass">)  [unwired: 8 in]
            n140 = Bundle By Name(cluster=w386, "SelfRef"=w382) -> (w387:T6)
            n141 = call <vilib>:"Add State(s) to Queue__jki_lib_state_machine.vi"("State(s) in (\"\")"=w390) -> ("States Out"=w389:string)  [unwired: 14 in]
          }
          frame "Instrument: Do Something" {
            # "communicate with\nhardware"
            n142 = Unbundle By Name(w401) -> ("SelfRef"=w400:refnum<class "Instrument.Framework-Template.lvclass">, "MessageToProcess.Message.Data"=w398:variant, "MessageToProcess.Message.ID"=w393:string)
            n143 = call "Instrument-Template.doSomethingExample.vi"("error in (no error)"=w399, "Data"=w398, "Instrument.Framework-Template in"=w400) -> ("error out"=w394:errorcluster, "Data out"=w392:variant, "Instrument.Framework-Template out"=w397:refnum<class "Instrument.Framework-Template.lvclass">)  [unwired: 6 in]
            n144 = Empty String/Path?(string/path=w392) -> (empty?=w391:bool)
            n145 = case shown="False" w391 {
              tunnel: w397 -> [w413 w415]
              tunnel: [w412 w415] -> w396
              tunnel: [w411 w414] -> w395
              tunnel: w392 -> [w409 _]
              tunnel: w394 -> [w408 w414]
              tunnel: w393 -> [w410 _]
              frame False {
                # "send data to\ninstrument:process.vi"
                n146 = call "enum to string.vim"("enum in"=Instrument.ProtectedCommands--Enum."setAllData" ("ProtectedCommands")) -> ("string out"=w406:string)  [unwired: 9 in, 1 out]
                n147 = call-poly <userlib>:"Instrument.sendMessageToProcess.vi"("ID"=w410, "error in (no error)"=w408, "Data"=w409, "Command"=w406, "Instrument"=w413) -> ("error out"=w411:errorcluster, "Instrument out"=w412:refnum<class "Instrument.Framework-Template.lvclass">)  [unwired: 5 in]
              }
              frame True {
              }
            }
            n148 = Bundle By Name(cluster=w401, "SelfRef"=w396) -> (w402:T6)
            n149 = call <vilib>:"Add State(s) to Queue__jki_lib_state_machine.vi"("State(s) in (\"\")"=w405) -> ("States Out"=w404:string)  [unwired: 14 in]
          }
          frame "Instrument: Log" {
            # "THIS process.vi is responsible for logging data. Logging can be triggered in the timeout (as shown in this template proces.vi's tieout case) OR it could be triggered by data changes, or any other way you can device.\n\nThe code above will log ALL data. But you have the ability to log a subset, log some items on a different schedule, etc."
            n150 = Unbundle By Name(w424) -> ("SelfRef"=w420:refnum<class "Instrument.Framework-Template.lvclass">)
            n151 = call-dynamic "Get SMO Database Paths.vi"("error in (no error)"=w417, "Instrument.Framework-Template in"=w420) -> ("error out"=w418:errorcluster, "Paths"=w421:string, "Instrument.Framework-Template out"=w416:refnum<class "Instrument.Framework-Template.lvclass">)  [unwired: 7 in]
            n152 = Unbundle By Name(w416) -> ("Data"=w419:T10)
            n153 = call <userlib>:"Instrument.logToDatabase.vi"("error in (no error)"=w418, "Data"=w419, "Paths"=w421, "Instrument"=w416) -> ("error out"=w422:errorcluster, "Instrument out"=w423:refnum<class "Instrument.Framework-Template.lvclass">)  [unwired: 6 in]
            n154 = Bundle By Name(cluster=w424, "SelfRef"=w423) -> (w425:T6)
            n155 = call <vilib>:"Add State(s) to Queue__jki_lib_state_machine.vi"("State(s) in (\"\")"=w428) -> ("States Out"=w427:string)  [unwired: 14 in]
          }
          frame "---------- Sequence ----------" {
            n156 = call <vilib>:"Add State(s) to Queue__jki_lib_state_machine.vi"("State(s) in (\"\")"=w433) -> ("States Out"=w432:string)  [unwired: 14 in]
          }
          frame "Sequence: Status" {
            # "Sequence: Status\n(Use this frame to pass the status to the UI, this VI's UI, etc)"
            n157 = call <vilib>:"Add State(s) to Queue__jki_lib_state_machine.vi"("State(s) in (\"\")"=w439) -> ("States Out"=w438:string)  [unwired: 14 in]
            "Status" <- w434
          }
          frame "Sequence: Wait" {
            # "Sequence: Wait\n(Non-Blocking Wait)"
            # "F = repeat this state. wait\nT = go to next state. don't wait"
            n158 = Unbundle By Name(w448) -> ("Running Step"=w441:i32)
            n159 = call <userlib>:"Wait Logic.vi"("error in (no error)"=w444, "Time"=w442) -> ("error out"=w443:errorcluster, "Status String"=w440:string, "Trigger"=w445:bool)  [unwired: 6 in, 1 out]
            n160 = Increment(x=w441) -> (x+1=w455:i32)
            n161 = Select(t=w455, s=w445, f=w441) -> (s? t:f=w446:i32)
            n162 = Select(t=u32 0, s=w445, f=u32 100 ("milliseconds to wait")) -> (s? t:f=w452:u32)
            n163 = call <userlib>:"Wait (ms)__ogtk.vi"("error in (no error)"=w443, "milliseconds to wait"=w452) -> ("error out"=w450:errorcluster)  [unwired: 8 in, 1 out]
            n164 = Bundle By Name(cluster=w448, "Running Step"=w446) -> (w447:T6)
            n165 = call <vilib>:"Build State String with Arguments__JKI_lib_State_Machine.vi"("Arguments (\"\")"=w440, "State"="Sequence: Status") -> ("State with Arguments"=w449:string)  [unwired: 4 in]
            n166 = call <vilib>:"Add State(s) to Queue__jki_lib_state_machine.vi"("State(s) in Front (\"\")"=w449, "State(s) in (\"\")"=w458) -> ("States Out"=w457:string)  [unwired: 13 in]
          }
        }
      }
    }
    frame Error {
    }
  }
  n167 = call-parent "Process.vi"("error in"=w5, "Instrument"=w4) -> ("error out"=w2:errorcluster, "Instrument out"=→"Instrument.Framework-Template out":refnum<class "Instrument.Framework-Template.lvclass">)  [unwired: 8 in]
  n168 = Merge Errors(w2, w1) -> (→"error out":errorcluster)
